vi "Cleanup (User).vi"(8 "error in":errorcluster, 11 "Node in":refnum<class "BLS Climate Chamber Template.lvclass">) -> (0 "error in":errorcluster, 3 "Node out":refnum<class "BLS Climate Chamber Template.lvclass">)   [LabVIEW 2023, in "BLS Climate Chamber Template.lvlib" / "BLS Climate Chamber Template.lvclass"]
uses:
  BLS Climate Chamber Template.lvclass
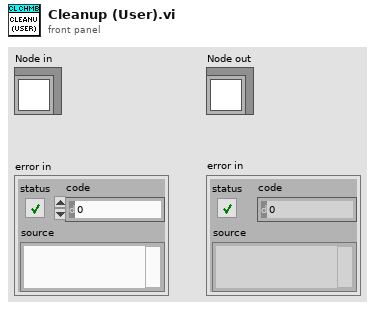
[diagram p1: front panel]
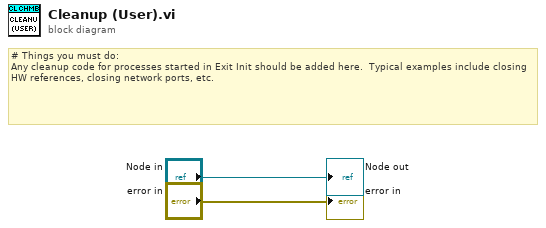
[diagram p0: block diagram]
diagram:
  # "# Things you must do:\nAny cleanup code for processes started in Exit Init should be added here.  Typical examples include closing HW references, closing network ports, etc."
  "Node out" <- "Node in"
  "error in" <- "error in"
